vi "Clear Subset (No Check).vi"(8 "error in (no error)":errorcluster, 9 "offset (0)":u64 format="%d bytes", 10 "length (-1: rest)":i64=-1 format="%d bytes", 11 "Pointer in":refnum<class "Pointer.lvclass">) -> (0 "error out":errorcluster, 3 "Pointer out":refnum<class "Pointer.lvclass">)   [LabVIEW 2017, in "Memory Manager.lvlib" / "Pointer.lvclass"]
doc: "Sets the subset of bytes specified by <b>offset</b> and <b>length</b> within the provided <b>pointer</b> to zero.\n\n<b>Note:</b> This VI is <b>unsafe</b>, meaning it does not performs null pointer and bounds checks to prevent invaid memory access. Invalid arguments provided to this method can crash or corrupt LabVIEW memory."
uses:
  Pointer.lvclass
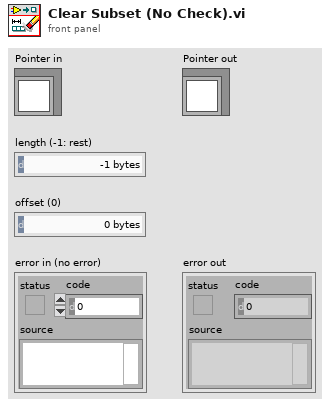
[diagram p1: front panel]
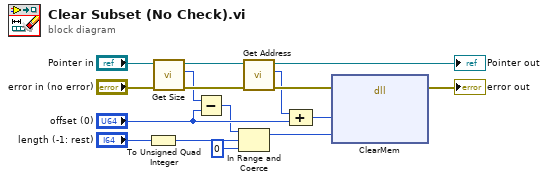
[diagram p0: block diagram]
diagram:
  n1 = To Unsigned Quad Integer(1:"length (-1: rest)") -> (0:w1:u64)
  n2 = call "Get Size.vi"("Pointer in"="Pointer in") -> ("size"=w2:u64, "Pointer out"=w4:refnum<class "Pointer.lvclass">)  [unwired: 9 in]
  n3 = Subtract(x=w2, y="offset (0)") -> (x-y=w3:u64)
  n4 = In Range and Coerce(upper limit=w3, x=w1, lower limit=u64 0) -> (coerced(x)=w6:u64)  [unwired: 1 out]
  n5 = call "Get Address.vi"("Pointer in"=w4) -> ("address"=w11:u64, "Pointer out"=→"Pointer out":refnum<class "Pointer.lvclass">)  [unwired: 9 in]
  n6 = Compound Arithmetic op=ADD(w11, "offset (0)") -> (w10:u64)
  n7 = dll-call lib="LabVIEW" fn="ClearMem"(error in="error in (no error)", "pointer"=w10, "size"=w6) -> (error out=→"error out":errorcluster)  [unwired: 5 in, 1 out]
